vi "Change State.vi"(8 "error in (no error)":errorcluster, 11 "Control Panel in":refnum<class "Control Panel.lvclass">) -> (0 "error out":errorcluster, 3 "Control Panel out":refnum<class "Control Panel.lvclass">)   [LabVIEW 2019, in "Control Panel.lvlib" / "Control Panel.lvclass"]
uses:
  Control Panel.lvclass
  Control Panel.lvclass/Control Panel.ctl
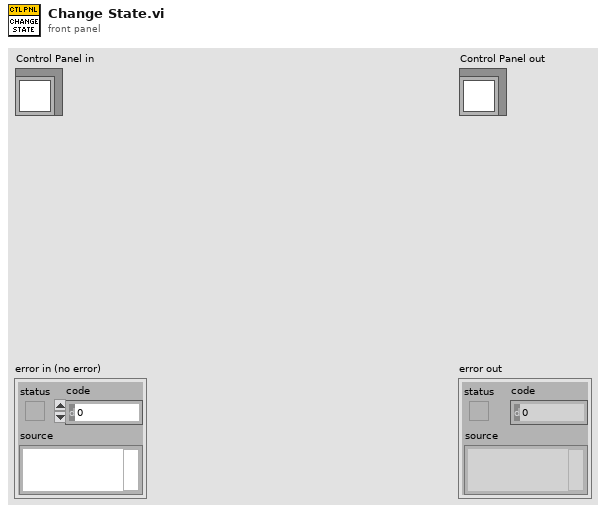
[diagram p1: front panel]
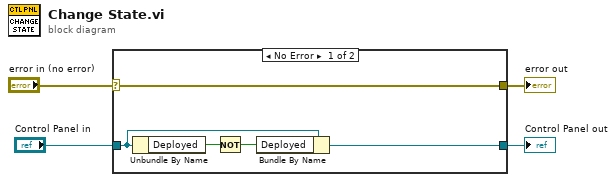
[diagram p0: block diagram]
diagram:
  n1 = case shown="No Error" "error in (no error)" {
    selector: "error in (no error)" -> [w9 w11]
    tunnel: [w9 w11] -> w3
    tunnel: [w7 w10] -> w1
    tunnel: "Control Panel in" -> [w8 w10]
    frame No Error {
      n2 = Unbundle By Name(w8) -> ("Deployed"=w6:bool)
      n3 = Not(x=w6) -> (.not. x?=w5:bool)
      n4 = Bundle By Name(cluster=w8, "Deployed"=w5) -> (w7:refnum<class "Control Panel.lvclass">)
    }
    frame Error {
    }
  }
  "error out" <- w3
  "Control Panel out" <- w1
